vi "2283_elevadorPID.vi"(8 "Tocando Switch abajo":bool, 9 "Tocando Switch Arriba":bool, 10 "process variable":dbl format="%.2f", 11 "setpoint":dbl format="%.2f") -> (2 "Output Elevador":dbl)   [LabVIEW 2014]
uses:
  <vilib>/addons/control/pid/pid.llb/PID (DBL).vi
  <vilib>/addons/control/pid/NI_PID_pid.lvlib
panel:
  in  "PID gains":T1={"proportional gain (Kc)"=0.035, "integral time (Ti, min)"=0.008, "derivative time (Td, min)"=0.0}
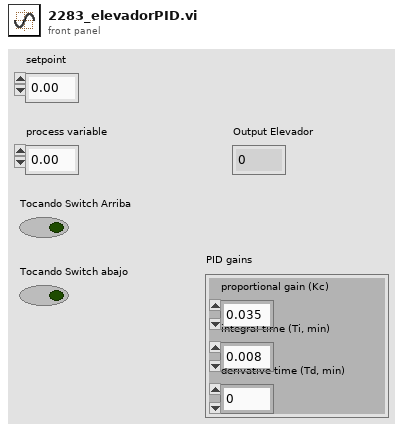
[diagram p1: front panel]
types:
  T1 = cluster{"proportional gain (Kc)":dbl, "integral time (Ti, min)":dbl, "derivative time (Td, min)":dbl}
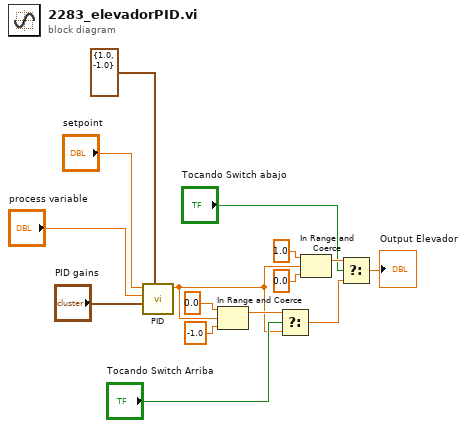
[diagram p0: block diagram]
diagram:
  n1 = call-poly <vilib>:"PID.vi"("output range"=cluster{"output high":dbl, "output low":dbl} {"output high"=1.0, "output low"=-1.0}, "PID gains"="PID gains", "process variable"="process variable", "setpoint"="setpoint") -> ("output"=w4:dbl)  [unwired: 6 in, 1 out]
  n2 = In Range and Coerce(upper limit=0.0, x=w4, lower limit=-1.0) -> (coerced(x)=w14:dbl)  [unwired: 1 out]
  n3 = Select(t=w14, s="Tocando Switch Arriba", f=w4) -> (s? t:f=w9:dbl)
  n4 = In Range and Coerce(upper limit=1.0, x=w4, lower limit=0.0) -> (coerced(x)=w11:dbl)  [unwired: 1 out]
  n5 = Select(t=w11, s="Tocando Switch abajo", f=w9) -> (s? t:f=→"Output Elevador":dbl)
